vi "B_calibration_stable.vi"() -> ()   [LabVIEW 2015]
doc: "Use this template to build a producer/consumer design pattern. Use this template when you need to execute a process, such as data analysis, when a data source, such as a triggered acquisition, produces data at an uneven rate and you need to execute the process when the data becomes available."
uses:
  <vilib>/Utility/file.llb/Write Delimited Spreadsheet (DBL).vi
panel:
  out "Coefficients":dbl[](array[numeric])
  out "B":dbl[](array[numeric])
  out "R":dbl[](array[numeric])
  out "XY Graph":cluster{dbl[], dbl[]}[](graph)
  out "B0 (T)":dbl
  out "B/V (T/V)":dbl
  out "I0 (A)":dbl
  out "V/I (Ohm)":dbl
  out "B_V":cluster{dbl[], "Best Linear Fit":dbl[]}[](graph)
  out "V_I":cluster{dbl[], "Best Linear Fit":dbl[]}[](graph)
  out "appended array":dbl[][](array[numeric])
  in  "dB":dbl=0.005
  in  "Dwell Time (ms)":u32=1
  in  "stop":bool
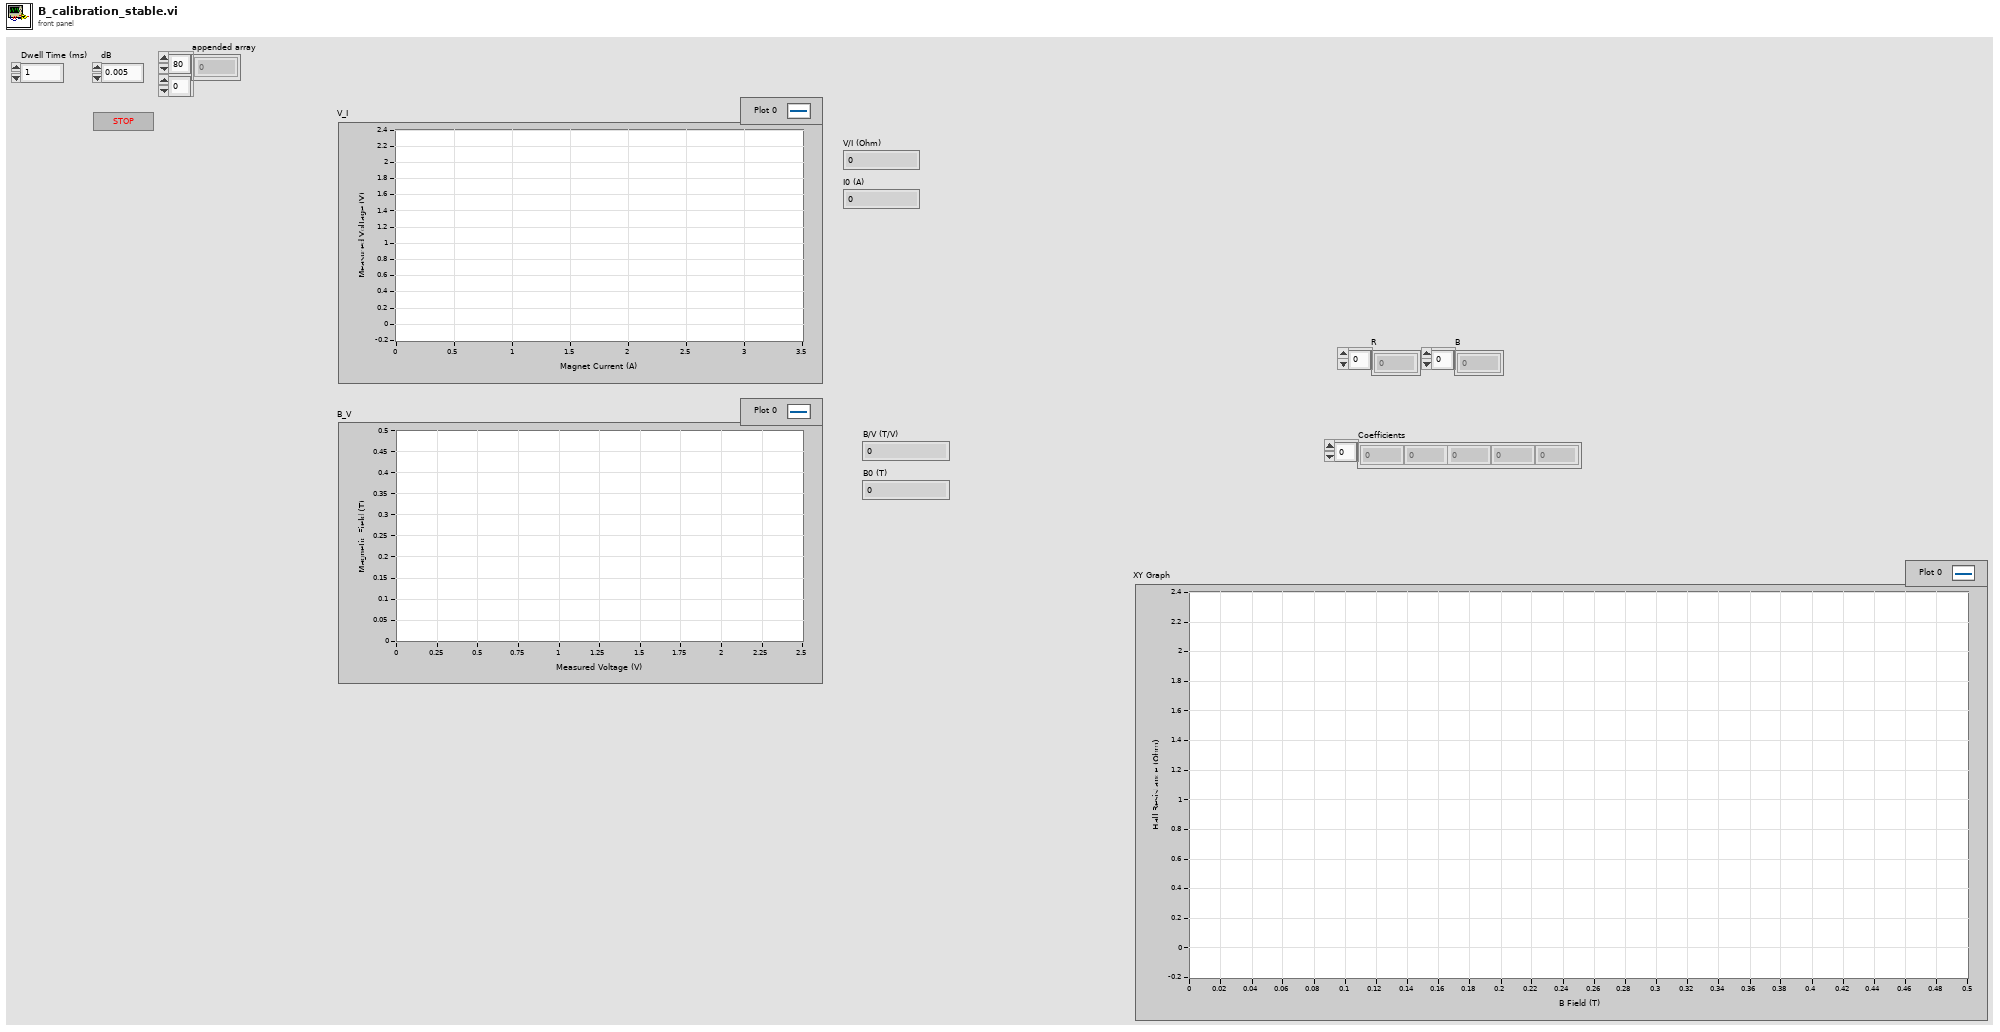
[diagram p1: front panel]
types:
  T1 = cluster{"I array out (A)":dbl[], "V array out (V)":dbl[]}
  T2 = cluster{"I array out (A)":dbl[], "Best Linear Fit":dbl[]}
  T3 = cluster{"V array out (V)":dbl[], "B array Out":dbl[]}
  T4 = cluster{"V array out (V)":dbl[], "Best Linear Fit 2":dbl[]}
  T5 = cluster{"I array out (A)":dbl[], "Best Linear Fit":dbl[]}[]
  T6 = cluster{"V array out (V)":dbl[], "Best Linear Fit 2":dbl[]}[]
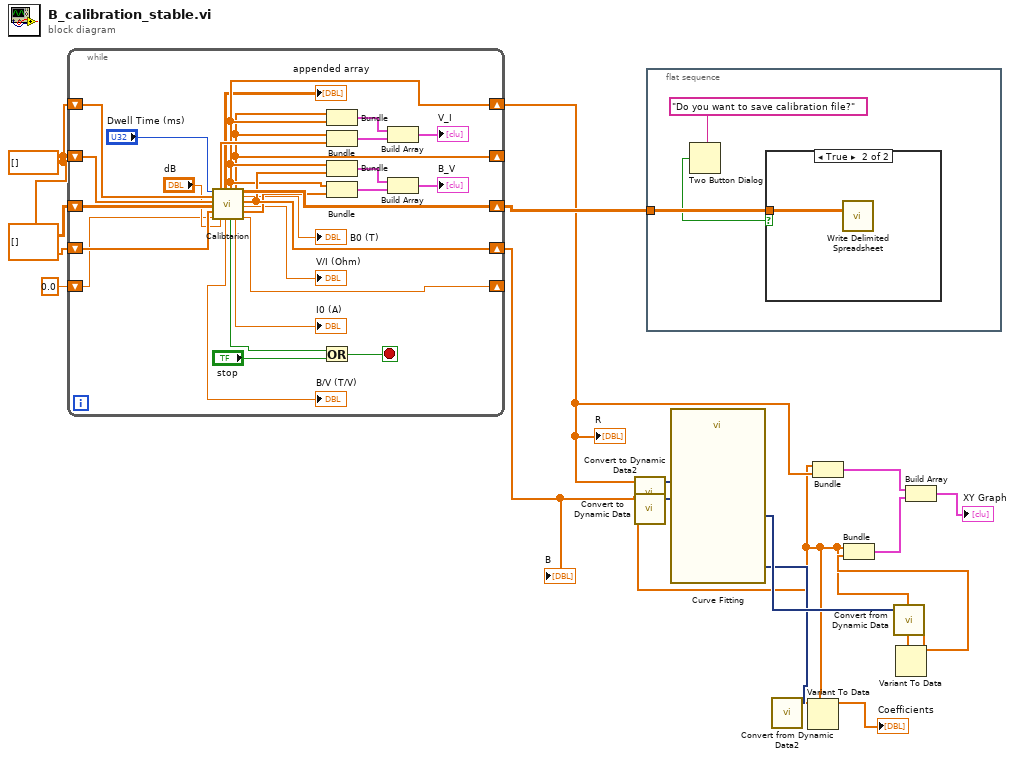
[diagram p0: block diagram]
diagram:
  w15 = dbl[] []
  n1 = while {
    shift-right: [w45] -> w17
    shift-left: dbl[][] [] -> [w44]
    shift-right: [w28] -> w5
    shift-left: w15 -> [w40]
    shift-right: [w37] -> w3
    shift-left: w15 -> [w39]
    shift-right: [w27] -> _
    shift-left: w15 -> [w38]
    shift-right: [w19] -> _
    shift-left: 0.0 ("Set Field out") -> [w18]
    stop <- w41 stop-if-true
    n2 = call "Calibtarion.vi"("Dwell Time (ms)"="Dwell Time (ms)", "V array in (V)"=w40, "I array in (A)"=w38, "Collected array in"=w44, "B array in (T)"=w39, "Set Field (T)"=w18, "dB"="dB") -> ("Best Linear Fit"=w29:dbl[], "appended array"=→"appended array":dbl[][], "slope"=→"B/V (T/V)":dbl, "V array out (V)"=w28:dbl[], "Boolean"=w43:bool, "I array out (A)"=w27:dbl[], "intercept 2"=→"I0 (A)":dbl, "Collected array out"=w45:dbl[][], "intercept"=→"B0 (T)":dbl, "B array Out"=w37:dbl[], "slope 2"=→"V/I (Ohm)":dbl, "Best Linear Fit 2"=w34:dbl[], "Set Field out"=w19:dbl)
    n3 = Or(x=w43, y="stop") -> (x .or. y?=w41:bool)
    n4 = Bundle("I array out (A)"=w27, "V array out (V)"=w28) -> (w36:T1)  [unwired: 1 in]
    n5 = Bundle("I array out (A)"=w27, "Best Linear Fit"=w29) -> (w30:T2)  [unwired: 1 in]
    n6 = Bundle("V array out (V)"=w28, "B array Out"=w37) -> (w32:T3)  [unwired: 1 in]
    n7 = Bundle("V array out (V)"=w28, "Best Linear Fit 2"=w34) -> (w33:T4)  [unwired: 1 in]
    n8 = Build Array(w36, w30) -> (→"V_I":T5)
    n9 = Build Array(w32, w33) -> (→"B_V":T6)
  }
  "R" <- w5
  "B" <- w3
  n10 = call "Convert to Dynamic Data2"("Array"=w5) -> ("Dynamic Data Type"=w12:dynamicdata)  [unwired: 3 in]
  n11 = call "Convert to Dynamic Data"("Array"=w3) -> ("Dynamic Data Type"=w13:dynamicdata)  [unwired: 3 in]
  n12 = flat-sequence {
    tunnel: w17 -> [w48]
    frame #0 {
      n13 = Two Button Dialog(message="Do you want to save calibration file?") -> (T button?=w47:bool)  [unwired: 2 in]
      n14 = case shown="True" w47 {
        tunnel: w48 -> [_ w49]
        frame False {
        }
        frame True {
          n15 = call-poly <vilib>:"Write Delimited Spreadsheet.vi"("2D data"=w49) -> ()  [unwired: 13 in, 2 out]
        }
      }
    }
  }
  n16 = call "Curve Fitting"("Locations"=w13, "Signals"=w12) -> ("best fit"=w10:dynamicdata, "polynomial coefficients"=w4:dynamicdata)  [unwired: 5 in, 3 out]
  n17 = call "Convert from Dynamic Data2"("Dynamic Data Type"=w4) -> ("Array"=w2:dbl[])  [unwired: 3 in]
  n18 = Variant To Data(type=w3, Variant=w2) -> (data=→"Coefficients":dbl[])  [unwired: 1 in, 1 out]
  n19 = Bundle(w3, w5) -> (w11:cluster{dbl[], dbl[]})  [unwired: 1 in]
  n20 = call "Convert from Dynamic Data"("Dynamic Data Type"=w10) -> ("Array"=w9:dbl[])  [unwired: 3 in]
  n21 = Variant To Data(type=w3, Variant=w9) -> (data=w8:dbl[])  [unwired: 1 in, 1 out]
  n22 = Bundle(w3, w8) -> (w7:cluster{dbl[], dbl[]})  [unwired: 1 in]
  n23 = Build Array(w11, w7) -> (→"XY Graph":cluster{dbl[], dbl[]}[])
